vi "eFGV - Cancel Log.vi"(6 "Action":T1, 8 "Error In":errorcluster, 11 "Cancel Log":bool) -> (0 "Error Out":errorcluster, 2 "Event Cancel Log":refnum<user-event>, 3 "Cancel Log Out":bool)   [LabVIEW 2020]
doc: "This eFGV used to trigger logging module delete the latest log file"
uses:
  Control/State - eFGV.ctl
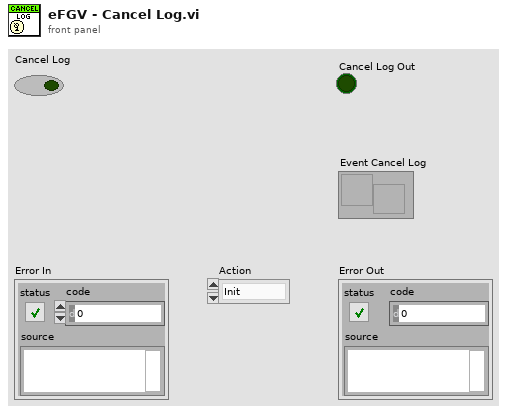
[diagram p1: front panel]
types:
  T1 = typedef "State - eFGV.ctl" = enum16{"Init", "Read", "Write", "Exit"}
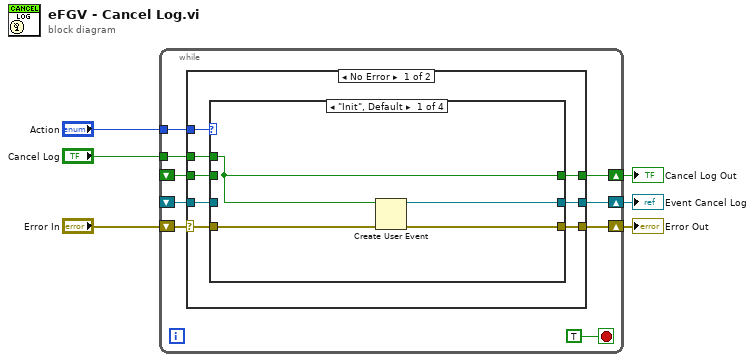
[diagram p0: block diagram]
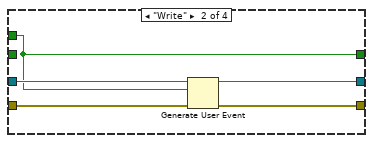
[diagram p2: hidden frame]
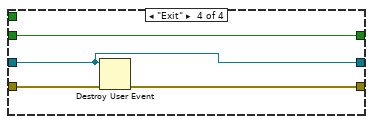
[diagram p4: hidden frame]
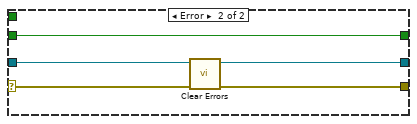
[diagram p5: hidden frame]
diagram:
  n1 = while {
    shift-right: [w14] -> w5
    shift-left: "Error In" -> [w15]
    tunnel: "Action" -> [w13]
    tunnel: "Cancel Log" -> [w11]
    shift-right: [w10] -> w1
    shift-left: _ -> [w8]
    shift-right: [w9] -> w2
    shift-left: _ -> [w7]
    stop <- TRUE stop-if-true
    n2 = case shown="No Error" w15 {
      selector: w15 -> [w23 w43]
      tunnel: w13 -> [w21 _]
      tunnel: w11 -> [w20 _]
      tunnel: [w22 w42] -> w14
      tunnel: [w19 w40] -> w10
      tunnel: [w18 w41] -> w9
      tunnel: w8 -> [w17 w40]
      tunnel: w7 -> [w16 w41]
      frame No Error {
        n3 = case shown="\"Init\", Default" w21 {
          tunnel: w20 -> [w24 w28 _ _]
          tunnel: w23 -> [w27 w32 w35 w39]
          tunnel: [w26 w31 w35 w38] -> w22
          tunnel: [w25 w30 w34 w37] -> w19
          tunnel: [w24 w28 w33 w36] -> w18
          tunnel: w17 -> [_ w29 w34 w37]
          tunnel: w16 -> [_ _ w33 w36]
          frame "Init", Default {
            n4 = Create User Event(user event datatype=w24, error in=w27) -> (user event=w25:refnum<user-event>, error out=w26:errorcluster)
          }
          frame "Write" {
            n5 = Generate User Event(user event=w29, event data cluster=w28, error in=w32) -> (user event out=w30:refnum<user-event>, error out=w31:errorcluster)  [unwired: 1 in]
          }
          frame "Read" {
          }
          frame "Exit" {
            n6 = Destroy User Event(user event=w37, error in=w39) -> (error out=w38:errorcluster)
          }
        }
      }
      frame Error {
        n7 = call <vilib>:"Clear Errors.vi"("error in (no error)"=w43) -> ("error out"=w42:errorcluster)  [unwired: 5 in, 1 out]
      }
    }
  }
  "Cancel Log Out" <- w2
  "Error Out" <- w5
  "Event Cancel Log" <- w1
